vi "all sensor graphbuffer.vi"(8 "Reset":bool, 9 "history length":u16=1000, 10 "WFGraph Refnum":refnum<vi>, 11 "Sensor Data":T1 {"Sensor array"."scaled" format="%.2f"; "Sensor array"."voltage" format="%.4f"; "Time" format="%<%I:%M:%S%2u %p\n%m/%d/%Y>T"}) -> (1 "data rate (Hz)":dbl format="%.2f", 2 "Mean":dbl[](array[numeric]) format="%.2f", 3 "Multiplot graph data":cluster{dbl[], dbl[]}[](array[cluster]) {"?" format="%.2f"; "?" format="%.2f"})   [LabVIEW 2012]
doc: "Takes an array containing one data point per channel and an arbitrary time. Creates data format required for an x-y plot with arbitrary data interval. Stores up to history number of data points per channel in a shift register.\nThis VI is reentrant meaning that it will hold different values if it is used at different places in a program. Thus more than one graph can be created!"
uses:
  TCP DAQ/Sensor data.ctl
  DAQ configuration/sensor cluster.ctl
  calibration/global scale array.vi
  <vilib>/Analysis/baseanly.llb/Mean (DBL).vi
  <vilib>/Analysis/NI_AALBase.lvlib
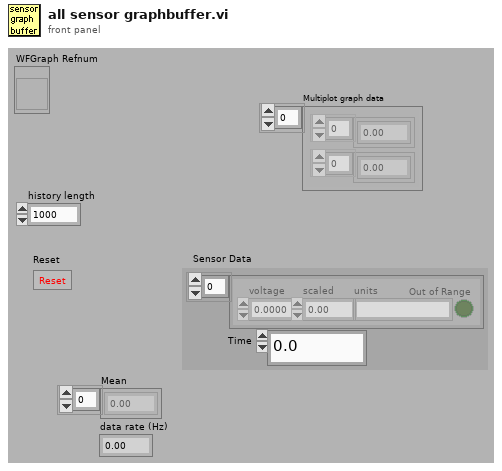
[diagram p1: front panel]
types:
  T1 = typedef "Sensor data.ctl" = cluster{" Sensor array":T2[], "Time":dbl}
  T2 = typedef "sensor cluster.ctl" = cluster{"voltage":sgl, "scaled":sgl, "units":string, "Out of Range":bool}
  T3 = typedef "calib array.ctl" = T4[]
  T4 = typedef "conversion.ctl" = cluster{"conversion matrix":sgl[][], "units":string, "name":string, "scale type":T5, "offset (volts)":dbl, "second channel":i8, "correspondence table":T6, "offset (physical units)":dbl, "pH scale":T7, "D.O.":T8}
  T5 = typedef "scale type.ctl" = enum16{"Volts", "Polynomial", "Correspondence Table", "pH", "Dissolved Oxygen", "Quadratic"}
  T6 = typedef "correspondence table.ctl" = cluster{"physical units":dbl, "volts":dbl}[]
  T7 = typedef "pH scale.ctl" = cluster{"Buffers":cluster{"Buffer":dbl, "Calibrated":bool, "V/T":dbl}[], "Temperature":dbl}
  T8 = typedef "DO scale.ctl" = cluster{"Temperature":dbl, "K":dbl, "barometric pressure":dbl}
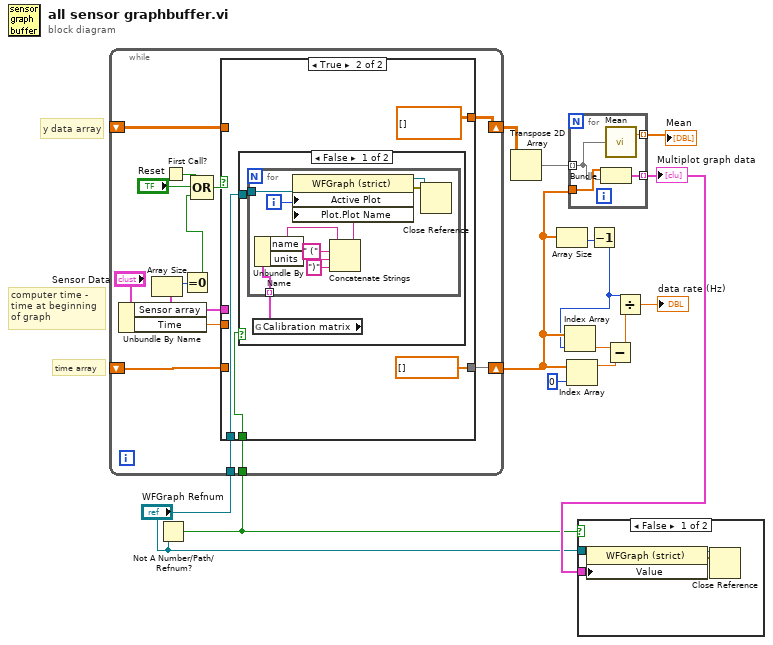
[diagram p0: block diagram]
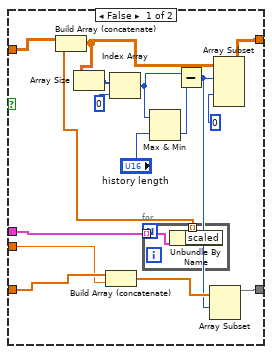
[diagram p3: hidden frame]
diagram:
  # "time array"
  # "y data array"
  # "computer time -  time at beginning of graph"
  n1 = Not A Number/Path/Refnum?(number/path/refnum="WFGraph Refnum") -> (NaN/Path/Refnum?=w1:bool)
  n2 = while {
    shift-left: _ -> [w27]
    shift-right: [w17] -> w10
    shift-left: _ -> [w29]
    shift-right: [w18] -> w14
    tunnel: "WFGraph Refnum" -> [w24]
    tunnel: w1 -> [w23]
    stop <- FALSE continue-if-true
    n3 = Unbundle By Name("Sensor Data") -> ("Sensor array"=w16:T2[], "Time"=w15:dbl)
    n4 = Array Size(array=w16) -> (size(s)=w20:i32)
    n5 = First Call?() -> (First Call?: T/F=w22:bool)
    n6 = Equal To 0?(x=w20) -> (x = 0?=w19:bool)
    n7 = Compound Arithmetic op=OR(w22, "Reset", w19) -> (w21:bool)
    n8 = case shown="True" w21 {
      tunnel: [w31 dbl[][] [] ("t")] -> w18
      tunnel: w29 -> [w35 _]
      tunnel: w27 -> [w34 _]
      tunnel: [w30 dbl[] []] -> w17
      tunnel: w24 -> [_ w49]
      tunnel: w23 -> [_ w48]
      tunnel: w16 -> [w33 _]
      tunnel: w15 -> [w32 _]
      frame False {
        n9 = Build Array (concatenate)(w34, w32) -> (w44:dbl[])
        n10 = for {
          tunnel: w33 -> [w47] mode=indexing
          tunnel: [w46] -> w45 mode=indexing
          n11 = Unbundle By Name(w47) -> ("scaled"=w46:sgl)
        }
        n12 = Build Array (concatenate)(w35, w45) -> (w36:dbl[][])
        n13 = Array Size(array=w36) -> (size(s)=w37:i32[])
        n14 = Index Array(array=w37, index=0 ("Index")) -> (element=w41:i32)
        n15 = Max & Min(x=w41, y="history length") -> (min(x,y)=w42:i32)  [unwired: 1 out]
        n16 = Subtract(x=w41, y=w42) -> (x-y=w43:i32)
        n17 = Array Subset(array=w44, index=w43) -> (w30:dbl[])  [unwired: 1 in]
        n18 = Array Subset(array=w36, index (row)=w43, index (col)=0 ("Array Index")) -> (w31:dbl[][])  [unwired: 2 in]
      }
      frame True {
        n19 = case shown="False" w48 {
          tunnel: w49 -> [w52 _]
          frame False {
            n20 = global read "global scale array.vi" "Calibration matrix"() -> (w53:T3)
            n21 = for {
              tunnel: w52 -> [w63]
              tunnel: w53 -> [w59] mode=indexing
              i -> [w62]
              n22 = Unbundle By Name(w59) -> ("name"=w58:string, "units"=w57:string)
              n23 = Concatenate Strings(w58, " (" ("string"), w57, ")" ("string")) -> (w54:string)
              n24 = property on="Property Node" class="WFGraph (strict)"(reference=w63, "Active Plot"=w62, "Plot.Plot Name"=w54) -> (reference out=w61:refnum<vi>, error out=w60:errorcluster)  [unwired: 1 in]
              n25 = Close Reference(reference=w61, error in (no error)=w60) -> ()  [unwired: 1 out]
            }
          }
          frame True {
          }
        }
      }
    }
  }
  n26 = Transpose 2D Array(2D array=w14) -> (transposed array=w12:dbl[][])
  n27 = Array Size(array=w10) -> (size(s)=w4:i32)
  n28 = Index Array(array=w10, index=0 ("Index")) -> (element=w7:dbl)
  n29 = for {
    tunnel: w12 -> [w65] mode=indexing
    tunnel: w10 -> [w67]
    tunnel: [w66] -> w13 mode=indexing
    tunnel: [w64] -> w11 mode=indexing
    n30 = Bundle(w67, w65) -> (w66:cluster{dbl[], dbl[]})  [unwired: 1 in]
    n31 = call-poly <vilib>:"Mean.vi"("X"=w65) -> ("mean"=w64:dbl)  [unwired: 1 out]
  }
  "Multiplot graph data" <- w13
  "Mean" <- w11
  n32 = case shown="False" w1 {
    tunnel: w13 -> [w71 _]
    tunnel: "WFGraph Refnum" -> [w68 _]
    frame False {
      n33 = property class="WFGraph (strict)"(reference=w68, "Value"=w71) -> (reference out=w69:refnum<vi>, error out=w70:errorcluster)  [unwired: 1 in]
      n34 = Close Reference(reference=w69, error in (no error)=w70) -> ()  [unwired: 1 out]
    }
    frame True {
    }
  }
  n35 = Decrement(x=w4) -> (x-1=w3:i32)
  n36 = Index Array(array=w10, index=w3) -> (element=w8:dbl)
  n37 = Subtract(x=w8, y=w7) -> (x-y=w6:dbl)
  n38 = Divide(x=w3, y=w6) -> (x/y=→"data rate (Hz)":dbl)
